vi "PlainTextToVariant (Standard).vi"(11 "String-formatted Value":string) -> (2 "Value Class":T1, 3 "Variant-formatted Value":variant)   [LabVIEW 2013, in "OpenSerializer.lvlib" / "Serializer.PlainText.lvclass"]
uses:
  Serializer.PlainText.lvclass
  Character Class -- Enum.ctl
  <vilib>/LabVIEW Open Source Project/Data Manipulation/Variant/Variant_EmptyCluster.vi
  <vilib>/Utility/GetType.llb/TD_Create Cluster.vi
  <vilib>/LabVIEW Open Source Project/Data Manipulation/Variant/OpenVariant.lvlib
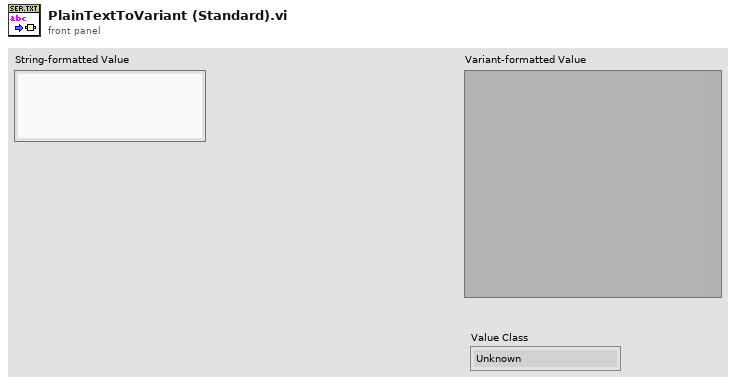
[diagram p1: front panel]
types:
  T1 = typedef "OpenSerializer.lvlib/Serializer.PlainText.lvclass/Character Class -- Enum.ctl" = enum16{"Unknown", "Sign", "Zero", "Integer", "Float", "Complex", "Scientific", "Engineering", "Hexadecimal", "Binary", "Decimal", "Octal", "Unit", "Invalid", "Timestamp", "Boolean", "String", "Path", "null", "cluster", "array"}
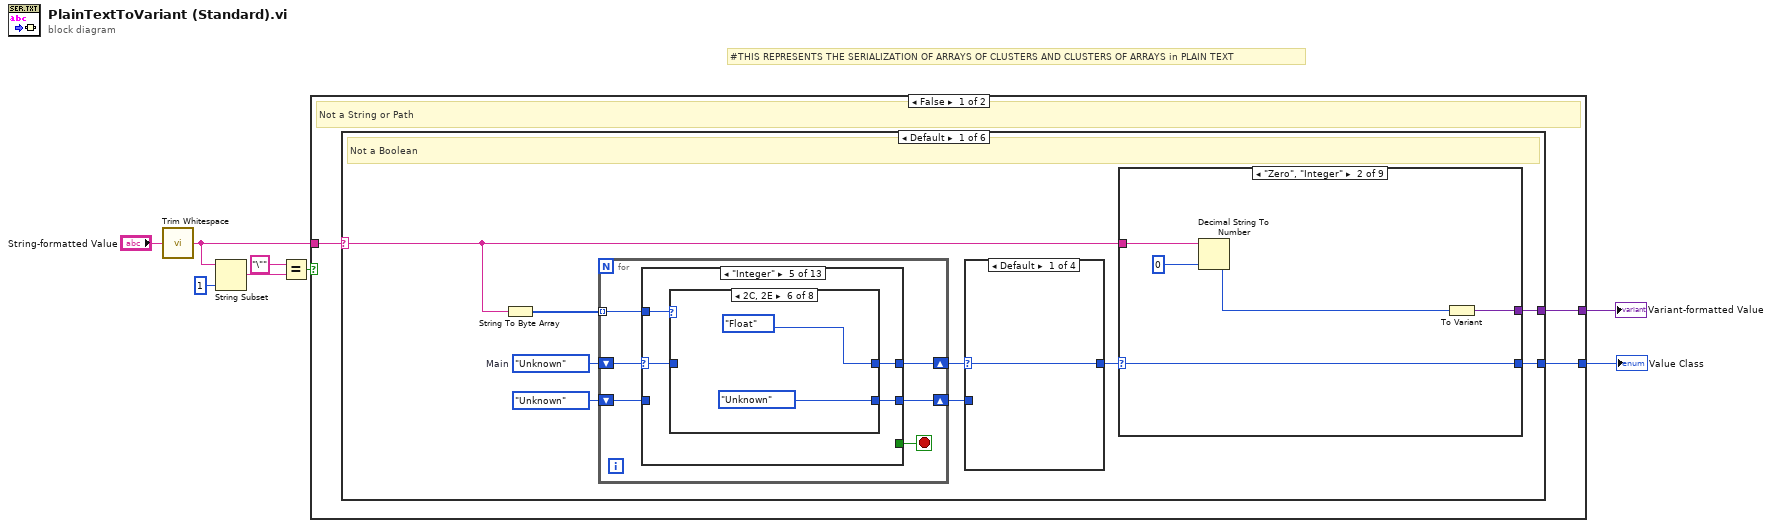
[diagram p0: block diagram]
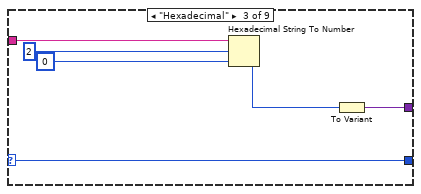
[diagram p3: hidden frame]
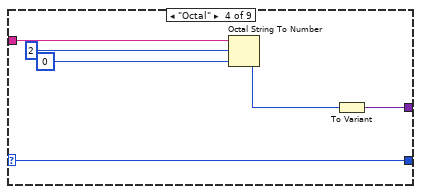
[diagram p4: hidden frame]
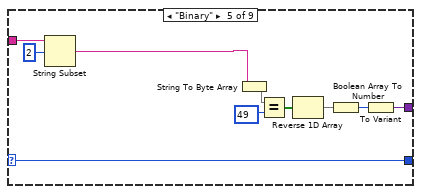
[diagram p5: hidden frame]
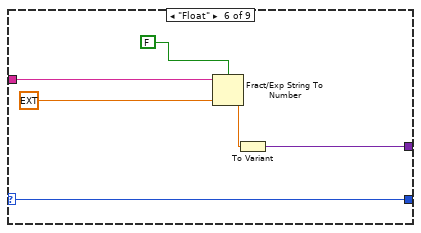
[diagram p6: hidden frame]
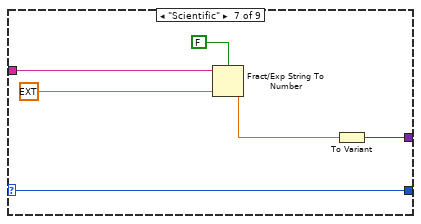
[diagram p7: hidden frame]
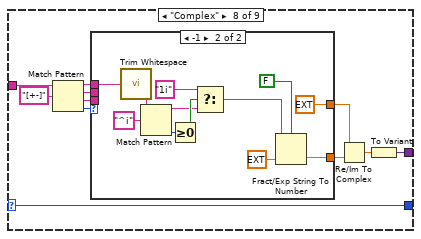
[diagram p8: hidden frame]
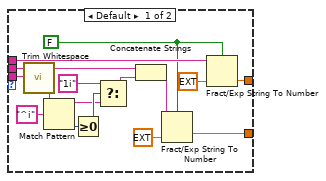
[diagram p9: hidden frame]
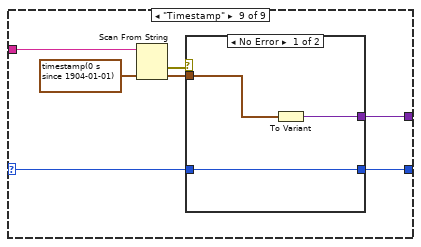
[diagram p10: hidden frame]
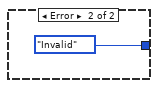
[diagram p11: hidden frame]
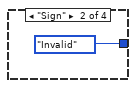
[diagram p12: hidden frame]
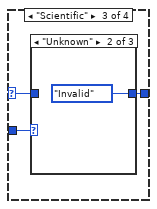
[diagram p13: hidden frame]
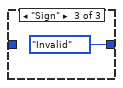
[diagram p15: hidden frame]
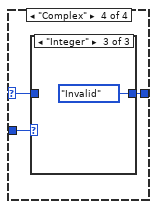
[diagram p16: hidden frame]
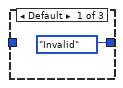
[diagram p17: hidden frame]
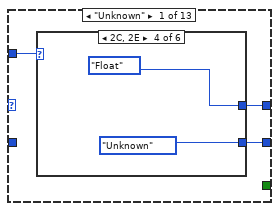
[diagram p19: hidden frame]
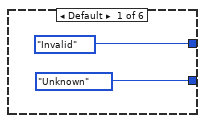
[diagram p20: hidden frame]
diagram:
  # "#THIS REPRESENTS THE SERIALIZATION OF ARRAYS OF CLUSTERS AND CLUSTERS OF ARRAYS in PLAIN TEXT"
  n1 = call <vilib>:"Trim Whitespace.vi"("string"="String-formatted Value") -> ("trimmed string"=w7:string)  [unwired: 1 in]
  n2 = String Subset(string=w7, length (rest)=1 ("length (rest)")) -> (substring=w5:string)  [unwired: 1 in]
  n3 = Equal?(x="\"", y=w5) -> (x = y?=w3:bool)
  n4 = case shown="False" w3 {
    tunnel: w7 -> [w11 w568]
    tunnel: [w10 w576] -> w8
    tunnel: [w9 w569] -> w2
    frame False {
      # "Not a String or Path"
      n5 = case shown="Default" w11 {
        selector: w11 -> [w15 _ _ _ w340 w457]
        tunnel: [w14 w328 w331 w335 w344 w461] -> w10
        tunnel: [w13 Character_Class_--_Enum."Boolean" Character_Class_--_Enum."Boolean" Character_Class_--_Enum."null" w343 w460] -> w9
        frame Default {
          w19 = Character_Class_--_Enum."Unknown"  # Main
          # "Not a Boolean"
          n6 = String To Byte Array(string=w15) -> (unsigned byte array=w20:u8[])
          n7 = for {
            tunnel: w20 -> [w129] mode=indexing
            shift-right: [w128] -> w18
            shift-left: w19 -> [w130]
            shift-right: [w126] -> w17
            shift-left: Character_Class_--_Enum."Unknown" -> [w127]
            stop <- w125 stop-if-true
            n8 = case shown="\"Integer\"" w130 {
              selector: w130 -> [_ w147 w150 w163 w188 w206 w212 w218 w224 w230 w233 w249 w289]
              tunnel: w129 -> [w133 _ w152 w165 w190 w208 w214 w220 w226 _ w235 w251 w291]
              tunnel: [w132 w147 w151 w164 w189 w207 w213 w219 w225 w230 w234 w250 w290] -> w128
              tunnel: w127 -> [_ w146 w148 _ _ _ _ _ _ _ _ w248 w288]
              tunnel: [w131 w146 w149 w162 w187 Character_Class_--_Enum."Unknown" Character_Class_--_Enum."Unknown" Character_Class_--_Enum."Unknown" Character_Class_--_Enum."Unknown" Character_Class_--_Enum."Unknown" w232 w247 w287] -> w126
              tunnel: [_ TRUE _ _ _ _ _ _ _ TRUE _ _ _] -> w125
              frame "Unknown" {
                n9 = case shown="2C, 2E" w133 {
                  tunnel: [Character_Class_--_Enum."Invalid" Character_Class_--_Enum."Sign" Character_Class_--_Enum."Integer" Character_Class_--_Enum."Float" Character_Class_--_Enum."Zero" w144] -> w132
                  tunnel: [Character_Class_--_Enum."Unknown" Character_Class_--_Enum."Unknown" Character_Class_--_Enum."Unknown" Character_Class_--_Enum."Unknown" Character_Class_--_Enum."Unknown" w144] -> w131
                  frame Default {
                  }
                  frame 43, 45 {
                  }
                  frame 49..57 {
                  }
                  frame 44, 46 {
                  }
                  frame 48 {
                  }
                  frame 105 {
                    w144 = Character_Class_--_Enum."Complex"
                  }
                }
              }
              frame "Invalid", Default {
              }
              frame "Sign" {
                n10 = case shown="2C, 2E" w152 {
                  tunnel: [Character_Class_--_Enum."Invalid" w156 Character_Class_--_Enum."Integer" w159 Character_Class_--_Enum."Float"] -> w151
                  tunnel: w150 -> [_ w156 _ _ _]
                  tunnel: [Character_Class_--_Enum."Unknown" w155 Character_Class_--_Enum."Unknown" w159 Character_Class_--_Enum."Unknown"] -> w149
                  tunnel: w148 -> [_ w155 _ _ _]
                  frame Default {
                  }
                  frame 32 {
                    # "space (ignore)"
                  }
                  frame 48..57 {
                  }
                  frame 105 {
                    w159 = Character_Class_--_Enum."Complex"
                  }
                  frame 44, 46 {
                  }
                }
              }
              frame "Zero" {
                n11 = case shown="Default" w165 {
                  tunnel: [Character_Class_--_Enum."Invalid" Character_Class_--_Enum."Integer" w171 Character_Class_--_Enum."Float" Character_Class_--_Enum."Hexadecimal" Character_Class_--_Enum."Binary" Character_Class_--_Enum."Octal" Character_Class_--_Enum."Decimal" w183 w184 Character_Class_--_Enum."Complex"] -> w164
                  tunnel: w163 -> [_ _ w171 _ _ _ _ _ w183 _ _]
                  tunnel: [Character_Class_--_Enum."Unknown" Character_Class_--_Enum."Unknown" Character_Class_--_Enum."Unknown" Character_Class_--_Enum."Unknown" Character_Class_--_Enum."Unknown" Character_Class_--_Enum."Unknown" Character_Class_--_Enum."Unknown" Character_Class_--_Enum."Unknown" Character_Class_--_Enum."Unknown" w184 Character_Class_--_Enum."Unknown"] -> w162
                  frame Default {
                  }
                  frame 49..57 {
                  }
                  frame 48 {
                  }
                  frame 44, 46 {
                  }
                  frame 120 {
                  }
                  frame 98 {
                  }
                  frame 111 {
                  }
                  frame 100 {
                  }
                  frame 32 {
                  }
                  frame 105 {
                    w184 = Character_Class_--_Enum."Complex"
                  }
                  frame 43, 45 {
                  }
                }
              }
              frame "Integer" {
                n12 = case shown="2C, 2E" w190 {
                  tunnel: [Character_Class_--_Enum."Invalid" w193 w194 w196 w198 Character_Class_--_Enum."Float" Character_Class_--_Enum."Complex" Character_Class_--_Enum."Scientific"] -> w189
                  tunnel: w188 -> [_ _ _ w196 w198 _ _ _]
                  tunnel: [Character_Class_--_Enum."Unknown" w193 w194 Character_Class_--_Enum."Unknown" Character_Class_--_Enum."Unknown" Character_Class_--_Enum."Unknown" Character_Class_--_Enum."Unknown" Character_Class_--_Enum."Unknown"] -> w187
                  frame Default {
                  }
                  frame 105 {
                    w193 = Character_Class_--_Enum."Complex"
                  }
                  frame 58 {
                    w194 = Character_Class_--_Enum."Timestamp"
                  }
                  frame 32 {
                  }
                  frame 48..57 {
                  }
                  frame 44, 46 {
                  }
                  frame 43, 45 {
                  }
                  frame 69, 101 {
                  }
                }
              }
              frame "Hexadecimal" {
                n13 = case shown="30..39, 41..46" w208 {
                  tunnel: [Character_Class_--_Enum."Invalid" w210] -> w207
                  tunnel: w206 -> [_ w210]
                  frame Default {
                  }
                  frame 48..57, 65..70 {
                  }
                }
              }
              frame "Decimal" {
                n14 = case shown="30..39" w214 {
                  tunnel: [Character_Class_--_Enum."Invalid" w216] -> w213
                  tunnel: w212 -> [_ w216]
                  frame Default {
                  }
                  frame 48..57 {
                  }
                }
              }
              frame "Octal" {
                n15 = case shown="30..37" w220 {
                  tunnel: [Character_Class_--_Enum."Invalid" w222] -> w219
                  tunnel: w218 -> [_ w222]
                  frame Default {
                  }
                  frame 48..55 {
                  }
                }
              }
              frame "Binary" {
                n16 = case shown="30, 31" w226 {
                  tunnel: [Character_Class_--_Enum."Invalid" w228] -> w225
                  tunnel: w224 -> [_ w228]
                  frame Default {
                  }
                  frame 48, 49 {
                  }
                }
              }
              frame "Timestamp" {
              }
              frame "Float" {
                n17 = case shown="2B, 2D" w235 {
                  tunnel: [Character_Class_--_Enum."Invalid" w239 Character_Class_--_Enum."Scientific" w243 Character_Class_--_Enum."Complex" w246] -> w234
                  tunnel: w233 -> [_ w239 _ w243 _ _]
                  tunnel: [Character_Class_--_Enum."Unknown" Character_Class_--_Enum."Unknown" Character_Class_--_Enum."Unknown" Character_Class_--_Enum."Unknown" Character_Class_--_Enum."Unknown" w246] -> w232
                  frame Default {
                  }
                  frame 48..57 {
                  }
                  frame 69, 101 {
                  }
                  frame 32 {
                  }
                  frame 43, 45 {
                  }
                  frame 105 {
                    w246 = Character_Class_--_Enum."Complex"
                  }
                }
              }
              frame "Scientific" {
                n18 = case shown="2B, 2D" w251 {
                  tunnel: [Character_Class_--_Enum."Invalid" w255 w267 w280] -> w250
                  tunnel: w249 -> [_ w254 w269 w282]
                  tunnel: w248 -> [w252 w256 w268 w281]
                  tunnel: [w252 w257 w270 w283] -> w247
                  frame Default {
                  }
                  frame 49..57 {
                    n19 = case shown="\"Unknown\"" w256 {
                      selector: w256 -> [_ _ _ w263 _]
                      tunnel: [w258 Character_Class_--_Enum."Integer" Character_Class_--_Enum."Integer" w263 Character_Class_--_Enum."Integer"] -> w257
                      tunnel: [w258 w259 w262 w264 w266] -> w255
                      tunnel: w254 -> [_ w259 w262 w264 w266]
                      frame Default {
                        w258 = Character_Class_--_Enum."Invalid"
                      }
                      frame "Sign" {
                      }
                      frame "Zero" {
                      }
                      frame "Integer" {
                      }
                      frame "Unknown" {
                      }
                    }
                  }
                  frame 48 {
                    n20 = case shown="\"Sign\"" w268 {
                      tunnel: [w271 Character_Class_--_Enum."Zero" Character_Class_--_Enum."Zero" Character_Class_--_Enum."Zero" Character_Class_--_Enum."Integer"] -> w270
                      tunnel: w269 -> [_ w272 w274 w276 w278]
                      tunnel: [w271 w272 w274 w276 w278] -> w267
                      frame Default {
                        w271 = Character_Class_--_Enum."Invalid"
                      }
                      frame "Unknown" {
                      }
                      frame "Sign" {
                      }
                      frame "Zero" {
                      }
                      frame "Integer" {
                      }
                    }
                  }
                  frame 43, 45 {
                    n21 = case shown="\"Unknown\"" w281 {
                      tunnel: [w284 Character_Class_--_Enum."Sign"] -> w283
                      tunnel: w282 -> [_ w285]
                      tunnel: [w284 w285] -> w280
                      frame Default {
                        w284 = Character_Class_--_Enum."Invalid"
                      }
                      frame "Unknown" {
                      }
                    }
                  }
                }
              }
              frame "Complex" {
                n22 = case shown="2C, 2E" w291 {
                  selector: w291 -> [_ _ _ w306 _]
                  tunnel: [w292 w294 w297 w309 w318] -> w290
                  tunnel: w289 -> [_ w294 w295 w307 w316]
                  tunnel: w288 -> [_ w293 w298 w310 w319]
                  tunnel: [w292 w293 w296 w308 w317] -> w287
                  frame Default {
                    w292 = Character_Class_--_Enum."Invalid"
                  }
                  frame 32 {
                  }
                  frame 48..57 {
                    n23 = case shown="Default" w298 {
                      selector: w298 -> [_ _ w302 w304]
                      tunnel: [w299 w301 w303 w305] -> w297
                      tunnel: [w299 Character_Class_--_Enum."Integer" w302 w304] -> w296
                      tunnel: w295 -> [_ w301 w303 w305]
                      frame Default {
                        w299 = Character_Class_--_Enum."Invalid"
                      }
                      frame "Unknown" {
                      }
                      frame "Integer" {
                      }
                      frame "Float" {
                      }
                    }
                  }
                  frame 44, 46 {
                    n24 = case shown="\"Unknown\"" w310 {
                      tunnel: [w311 w313 w315] -> w309
                      tunnel: [w311 Character_Class_--_Enum."Float" Character_Class_--_Enum."Float"] -> w308
                      tunnel: w307 -> [_ w313 w315]
                      tunnel: w306 -> [_ _ _]
                      frame Default {
                        w311 = Character_Class_--_Enum."Invalid"
                      }
                      frame "Unknown" {
                      }
                      frame "Integer" {
                      }
                    }
                  }
                  frame 105 {
                    n25 = case shown="\"Float\"" w319 {
                      tunnel: [w320 w322 w324 w326] -> w318
                      tunnel: [w320 Character_Class_--_Enum."Complex" Character_Class_--_Enum."Complex" Character_Class_--_Enum."Complex"] -> w317
                      tunnel: w316 -> [_ w322 w324 w326]
                      frame Default {
                        w320 = Character_Class_--_Enum."Invalid"
                      }
                      frame "Unknown" {
                      }
                      frame "Integer" {
                      }
                      frame "Float" {
                      }
                    }
                  }
                }
              }
            }
          }
          n26 = case shown="Default" w18 {
            selector: w18 -> [w111 _ w113 w119]
            tunnel: w17 -> [_ _ w115 w121]
            tunnel: [w111 Character_Class_--_Enum."Invalid" w114 w120] -> w16
            frame Default {
            }
            frame "Sign" {
            }
            frame "Scientific" {
              n27 = case shown="\"Unknown\"" w115 {
                tunnel: [w116 Character_Class_--_Enum."Invalid" Character_Class_--_Enum."Invalid"] -> w114
                tunnel: w113 -> [w116 _ _]
                frame Default {
                }
                frame "Unknown" {
                }
                frame "Sign" {
                }
              }
            }
            frame "Complex" {
              n28 = case shown="\"Integer\"" w121 {
                tunnel: [Character_Class_--_Enum."Invalid" w123 Character_Class_--_Enum."Invalid" ("Main")] -> w120
                tunnel: w119 -> [_ w123 _]
                frame Default {
                }
                frame "Complex" {
                }
                frame "Integer" {
                }
              }
            }
          }
          n29 = case shown="\"Zero\", \"Integer\"" w16 {
            selector: w16 -> [w21 w22 w27 w33 w39 w50 w56 w70 w100]
            tunnel: w15 -> [_ w26 w32 w38 w47 w54 w60 w66 w106]
            tunnel: [_ w23 w29 w35 w48 w51 w57 w71 w103] -> w14
            tunnel: [w21 w22 w27 w33 w39 w50 w56 w70 w101] -> w13
            frame Default {
            }
            frame "Zero", "Integer" {
              n30 = Decimal String To Number(string=w26, default (0L)=i64 0 ("default (0 I32)")) -> (number=w24:i64)  [unwired: 1 in, 1 out]
              n31 = To Variant(anything=w24) -> (Variant=w23:variant)
            }
            frame "Hexadecimal" {
              n32 = Hexadecimal String To Number(string=w32, offset=2, default (0uL)=i64 0 ("default (0 I32)")) -> (number=w30:i64)  [unwired: 1 out]
              n33 = To Variant(anything=w30) -> (Variant=w29:variant)
            }
            frame "Octal" {
              n34 = Octal String To Number(2:i64 0 ("default (0 I32)"), 3:2 ("offset"), 4:w38) -> (0:w36:i64)  [unwired: 1 out]
              n35 = To Variant(anything=w36) -> (Variant=w35:variant)
            }
            frame "Binary" {
              n36 = String Subset(string=w47, offset (0)=2) -> (substring=w45:string)  [unwired: 1 in]
              n37 = String To Byte Array(string=w45) -> (unsigned byte array=w43:u8[])
              n38 = Equal?(x=w43, y=u8 49 ("offset (0)")) -> (x = y?=w42:bool[])
              n39 = Reverse 1D Array(array=w42) -> (reversed array=w40:bool[])
              n40 = Boolean Array To Number(Boolean array=w40) -> (number=w44:u32)
              n41 = To Variant(anything=w44) -> (Variant=w48:variant)
            }
            frame "Float" {
              n42 = Fract/Exp String To Number(use system decimal point (T)=FALSE, string=w54, default (0 dbl)=ext 0.0 ("default (0 I32)")) -> (number=w52:ext)  [unwired: 1 in, 1 out]
              n43 = To Variant(anything=w52) -> (Variant=w51:variant)
            }
            frame "Scientific" {
              n44 = Fract/Exp String To Number(use system decimal point (T)=FALSE, string=w60, default (0 dbl)=ext 0.0 ("default (0 I32)")) -> (number=w58:ext)  [unwired: 1 in, 1 out]
              n45 = To Variant(anything=w58) -> (Variant=w57:variant)
            }
            frame "Complex" {
              n46 = Match Pattern(string=w66, regular expression="[+-]") -> (before substring=w63:string, match substring=w61:string, after substring=w62:string, offset past match=w67:i32)  [unwired: 1 in]
              n47 = case shown="-1" w67 {
                tunnel: [w84 ext 0.0 ("default (0 DBL)")] -> w64
                tunnel: [w86 w97] -> w65
                tunnel: w63 -> [w83 w90]
                tunnel: w62 -> [w74 _]
                tunnel: w61 -> [w77 _]
                frame Default {
                  w72 = FALSE ("use system decimal point (T)")
                  n48 = call <vilib>:"Trim Whitespace.vi"("string"=w74) -> ("trimmed string"=w75:string)  [unwired: 1 in]
                  n49 = Match Pattern(string=w75, regular expression="^i") -> (before substring=w80:string, offset past match=w82:i32)  [unwired: 1 in, 2 out]
                  n50 = Greater Or Equal To 0?(x=w82) -> (x >= 0?=w81:bool)
                  n51 = Select(t="1i", s=w81, f=w80) -> (s? t:f=w78:string)
                  n52 = Concatenate Strings(w77, w78) -> (w76:string)
                  n53 = Fract/Exp String To Number(use system decimal point (T)=w72, string=w76, default (0 dbl)=ext 0.0 ("default (0 DBL)")) -> (number=w86:ext)  [unwired: 1 in, 1 out]
                  n54 = Fract/Exp String To Number(use system decimal point (T)=w72, string=w83, default (0 dbl)=ext 0.0 ("default (0 DBL)")) -> (number=w84:ext)  [unwired: 1 in, 1 out]
                }
                frame -1 {
                  n55 = call <vilib>:"Trim Whitespace.vi"("string"=w90) -> ("trimmed string"=w92:string)  [unwired: 1 in]
                  n56 = Match Pattern(string=w92, regular expression="^i") -> (before substring=w94:string, offset past match=w96:i32)  [unwired: 1 in, 2 out]
                  n57 = Greater Or Equal To 0?(x=w96) -> (x >= 0?=w95:bool)
                  n58 = Select(t="1i", s=w95, f=w94) -> (s? t:f=w89:string)
                  n59 = Fract/Exp String To Number(use system decimal point (T)=FALSE, string=w89, default (0 dbl)=ext 0.0 ("default (0 DBL)")) -> (number=w97:ext)  [unwired: 1 in, 1 out]
                }
              }
              n60 = Re/Im To Complex(1:w65, 2:w64) -> (0:w69:cxt)
              n61 = To Variant(anything=w69) -> (Variant=w71:variant)
            }
            frame "Timestamp" {
              n62 = Scan From String(input string=w106, default 1=timestamp(0 s since 1904-01-01)) -> (error out=w102:errorcluster, output 1=w104:timestamp)  [unwired: 3 in, 2 out]
              n63 = case shown="No Error" w102 {
                tunnel: w104 -> [w109 _]
                tunnel: [w108 _] -> w103
                tunnel: [w107 Character_Class_--_Enum."Invalid"] -> w101
                tunnel: w100 -> [w107 _]
                frame No Error {
                  n64 = To Variant(anything=w109) -> (Variant=w108:variant)
                }
                frame Error {
                }
              }
            }
          }
        }
        frame "true" {
          # "BOOLEAN (TRUE)"
          n65 = To Variant(anything=TRUE) -> (Variant=w328:variant)
        }
        frame "false" {
          # "BOOLEAN (FALSE)"
          n66 = To Variant(anything=FALSE) -> (Variant=w331:variant)
        }
        frame "null" {
          # "null"
          n67 = To Variant(anything=variant ("variant")) -> (Variant=w335:variant)
        }
        frame "{".."{~" {
          # "cluster"
          n68 = String Length(string=w340) -> (length=w342:i32)
          n69 = Subtract(x=w342, y=1) -> (x-y=w336:i32)
          n70 = String Subset(string=w340, offset (0)=w336) -> (substring=w338:string)  [unwired: 1 in]
          n71 = Equal?(x="}", y=w338) -> (x = y?=w337:bool)
          n72 = case shown="True" w337 {
            tunnel: [w353 w452] -> w344
            tunnel: [Character_Class_--_Enum."cluster" Character_Class_--_Enum."Invalid"] -> w343
            tunnel: w340 -> [w359 _]
            tunnel: w336 -> [w357 _]
            frame True {
              n73 = Decrement(x=w357) -> (x-1=w356:i32)
              n74 = String Subset(string=w359, offset (0)=1, length (rest)=w356) -> (substring=w355:string)
              n75 = call <vilib>:"Trim Whitespace.vi"("string"=w355) -> ("trimmed string"=w350:string)  [unwired: 1 in]
              n76 = String Length(string=w350) -> (length=w351:i32)
              n77 = for {
                N: w351 -> [_]
                shift-right: [w364] -> w347
                shift-left: string[] [] -> [w365]
                tunnel: w350 -> [w370]
                shift-right: [w363] -> w348
                shift-left: "" -> [w366]
                shift-right: [w361] -> _
                shift-left: Character_Class_--_Enum."Unknown" -> [w362]
                i -> [w369]
                n78 = String Subset(string=w370, offset (0)=w369, length (rest)=1 ("offset (0)")) -> (substring=w367:string)
                n79 = case shown="Default" w367 {
                  selector: w367 -> [w374 w377 w395 w407 w421 w435]
                  tunnel: w366 -> [w373 w382 w396 w408 w422 w436]
                  tunnel: w365 -> [w375 w381 w398 w410 w424 w438]
                  tunnel: [w375 w380 w398 w410 w424 w438] -> w364
                  tunnel: [w372 w379 w394 w406 w420 w434] -> w363
                  tunnel: w362 -> [w371 w378 w397 w409 w423 w437]
                  tunnel: [w371 w376 w393 w405 w419 w433] -> w361
                  frame Default {
                    n80 = Concatenate Strings(w373, w374) -> (w372:string)
                  }
                  frame "," {
                    n81 = case shown="\"Unknown\", Default" w378 {
                      selector: w378 -> [w383 w388]
                      tunnel: w382 -> [w387 w391]
                      tunnel: w381 -> [w386 w392]
                      tunnel: [w385 w392] -> w380
                      tunnel: ["" w389] -> w379
                      tunnel: w377 -> [_ w390]
                      tunnel: [w383 w388] -> w376
                      frame "Unknown", Default {
                        n82 = Build Array (concatenate)(w386, w387) -> (w385:string[])
                      }
                      frame "cluster", "array" {
                        n83 = Concatenate Strings(w391, w390) -> (w389:string)
                      }
                    }
                  }
                  frame "{" {
                    n84 = case shown="Default" w397 {
                      selector: w397 -> [_ w401]
                      tunnel: w396 -> [_ w404]
                      tunnel: w395 -> [w399 w403]
                      tunnel: [w399 w402] -> w394
                      tunnel: [Character_Class_--_Enum."cluster" w401] -> w393
                      frame Default {
                      }
                      frame "cluster" {
                        n85 = Concatenate Strings(w404, w403) -> (w402:string)
                      }
                    }
                  }
                  frame "}" {
                    n86 = case shown="\"cluster\"" w409 {
                      selector: w409 -> [w411 _]
                      tunnel: w408 -> [w414 w416]
                      tunnel: w407 -> [w413 w417]
                      tunnel: [w412 w415] -> w406
                      tunnel: [w411 Character_Class_--_Enum."Unknown"] -> w405
                      frame Default {
                        n87 = Concatenate Strings(w414, w413) -> (w412:string)
                      }
                      frame "cluster" {
                        n88 = Concatenate Strings(w416, w417) -> (w415:string)
                      }
                    }
                  }
                  frame "[" {
                    n89 = case shown="Default" w423 {
                      tunnel: w422 -> [w428 w430]
                      tunnel: w421 -> [w427 w431]
                      tunnel: [w426 w429] -> w420
                      tunnel: [Character_Class_--_Enum."array" Character_Class_--_Enum."array"] -> w419
                      frame Default {
                        n90 = Concatenate Strings(w428, w427) -> (w426:string)
                      }
                      frame "cluster" {
                        n91 = Concatenate Strings(w430, w431) -> (w429:string)
                      }
                    }
                  }
                  frame "]" {
                    n92 = case shown="\"array\"" w437 {
                      selector: w437 -> [w439 _]
                      tunnel: w436 -> [w442 w444]
                      tunnel: w435 -> [w441 w445]
                      tunnel: [w440 w443] -> w434
                      tunnel: [w439 Character_Class_--_Enum."Unknown"] -> w433
                      frame Default {
                        n93 = Concatenate Strings(w442, w441) -> (w440:string)
                      }
                      frame "array" {
                        n94 = Concatenate Strings(w444, w445) -> (w443:string)
                      }
                    }
                  }
                }
              }
              n95 = Build Array (concatenate)(w347, w348) -> (w346:string[])
              n96 = for {
                tunnel: w346 -> [w449] mode=indexing
                tunnel: [w447] -> w354 mode=indexing
                n97 = call <vilib>:"Trim Whitespace.vi"("string"=w449) -> ("trimmed string"=w448:string)  [unwired: 1 in]
                n98 = call "PlainTextToVariant (Standard).vi"("String-formatted Value"=w448) -> ("Variant-formatted Value"=w447:variant)  [unwired: 9 in, 1 out]
              }
              n99 = call <vilib>:"Variant_BuildClusterFromElementArray.vi"("Elements"=w354) -> ("Cluster"=w353:variant)  [unwired: 10 in]
            }
            frame False {
              n100 = To Variant(anything=variant ("variant")) -> (Variant=w452:variant)
            }
          }
        }
        frame "[".."[~" {
          # "array"
          n101 = String Length(string=w457) -> (length=w459:i32)
          n102 = Subtract(x=w459, y=1) -> (x-y=w453:i32)
          n103 = String Subset(string=w457, offset (0)=w453) -> (substring=w455:string)  [unwired: 1 in]
          n104 = Equal?(x="]", y=w455) -> (x = y?=w454:bool)
          n105 = case shown="True" w454 {
            tunnel: [w465 w567] -> w461
            tunnel: [Character_Class_--_Enum."array" Character_Class_--_Enum."Invalid"] -> w460
            tunnel: w457 -> [w463 _]
            tunnel: w453 -> [w475 _]
            frame True {
              # "#THIS IS UPDATED AS WELL\nto support undefined array input"
              n106 = Decrement(x=w475) -> (x-1=w474:i32)
              n107 = String Subset(string=w463, offset (0)=1, length (rest)=w474) -> (substring=w462:string)
              n108 = call <vilib>:"Trim Whitespace.vi"("string"=w462) -> ("trimmed string"=w471:string)  [unwired: 1 in]
              n109 = String Length(string=w471) -> (length=w472:i32)
              n110 = for {
                N: w472 -> [_]
                shift-right: [w481] -> w468
                shift-left: string[] [] -> [w482]
                tunnel: w471 -> [w487]
                shift-right: [w480] -> w469
                shift-left: "" -> [w483]
                shift-right: [w478] -> _
                shift-left: Character_Class_--_Enum."Unknown" -> [w479]
                i -> [w486]
                n111 = String Subset(string=w487, offset (0)=w486, length (rest)=1 ("offset (0)")) -> (substring=w484:string)
                n112 = case shown="\"]\"" w484 {
                  selector: w484 -> [w491 w494 w512 w524 w536 w550]
                  tunnel: w483 -> [w490 w499 w513 w525 w537 w551]
                  tunnel: w482 -> [w492 w498 w515 w527 w539 w553]
                  tunnel: [w492 w497 w515 w527 w539 w553] -> w481
                  tunnel: [w489 w496 w511 w523 w535 w549] -> w480
                  tunnel: w479 -> [w488 w495 w514 w526 w538 w552]
                  tunnel: [w488 w493 w510 w522 w534 w548] -> w478
                  frame Default {
                    n113 = Concatenate Strings(w490, w491) -> (w489:string)
                  }
                  frame "," {
                    n114 = case shown="\"cluster\"" w495 {
                      selector: w495 -> [w500 w505]
                      tunnel: w499 -> [w504 w508]
                      tunnel: w498 -> [w503 w509]
                      tunnel: [w502 w509] -> w497
                      tunnel: ["" w506] -> w496
                      tunnel: w494 -> [_ w507]
                      tunnel: [w500 w505] -> w493
                      frame "Unknown", Default {
                        n115 = Build Array (concatenate)(w503, w504) -> (w502:string[])
                      }
                      frame "cluster" {
                        n116 = Concatenate Strings(w508, w507) -> (w506:string)
                      }
                    }
                  }
                  frame "[" {
                    n117 = case shown="\"array\"" w514 {
                      selector: w514 -> [_ w518]
                      tunnel: w513 -> [_ w521]
                      tunnel: w512 -> [w516 w520]
                      tunnel: [w516 w519] -> w511
                      tunnel: [Character_Class_--_Enum."array" w518] -> w510
                      frame Default {
                      }
                      frame "array" {
                        n118 = Concatenate Strings(w521, w520) -> (w519:string)
                      }
                    }
                  }
                  frame "{" {
                    n119 = case shown="Default" w526 {
                      selector: w526 -> [_ w530]
                      tunnel: w525 -> [_ w533]
                      tunnel: w524 -> [w528 w532]
                      tunnel: [w528 w531] -> w523
                      tunnel: [Character_Class_--_Enum."cluster" w530] -> w522
                      frame Default {
                      }
                      frame "cluster" {
                        n120 = Concatenate Strings(w533, w532) -> (w531:string)
                      }
                    }
                  }
                  frame "]" {
                    n121 = case shown="\"array\"" w538 {
                      selector: w538 -> [w540 _]
                      tunnel: w537 -> [w543 w545]
                      tunnel: w536 -> [w542 w546]
                      tunnel: [w541 w544] -> w535
                      tunnel: [w540 Character_Class_--_Enum."Unknown"] -> w534
                      frame Default {
                        n122 = Concatenate Strings(w543, w542) -> (w541:string)
                      }
                      frame "array" {
                        n123 = Concatenate Strings(w545, w546) -> (w544:string)
                      }
                    }
                  }
                  frame "}" {
                    n124 = case shown="\"cluster\"" w552 {
                      selector: w552 -> [w554 _]
                      tunnel: w551 -> [w557 w559]
                      tunnel: w550 -> [w556 w560]
                      tunnel: [w555 w558] -> w549
                      tunnel: [w554 Character_Class_--_Enum."Unknown"] -> w548
                      frame Default {
                        n125 = Concatenate Strings(w557, w556) -> (w555:string)
                      }
                      frame "cluster" {
                        n126 = Concatenate Strings(w559, w560) -> (w558:string)
                      }
                    }
                  }
                }
              }
              n127 = Build Array (concatenate)(w468, w469) -> (w467:string[])
              n128 = for {
                tunnel: w467 -> [w564] mode=indexing
                tunnel: [w562] -> w464 mode=indexing
                n129 = call <vilib>:"Trim Whitespace.vi"("string"=w564) -> ("trimmed string"=w563:string)  [unwired: 1 in]
                n130 = call "PlainTextToVariant (Standard).vi"("String-formatted Value"=w563) -> ("Variant-formatted Value"=w562:variant)  [unwired: 9 in, 1 out]
              }
              n131 = call <vilib>:"Variant_BuildArrayFromElementArray.vi"("Elements"=w464) -> ("Output Array"=w465:variant)  [unwired: 9 in, 1 out]
            }
            frame False {
              n132 = To Variant(anything=variant ("variant")) -> (Variant=w567:variant)
            }
          }
        }
      }
    }
    frame True {
      # "String or Path"
      n133 = String Length(string=w568) -> (length=w575:i32)
      n134 = Decrement(x=w575) -> (x-1=w571:i32)
      n135 = String Subset(string=w568, offset (0)=w571, length (rest)=1 ("length (rest)")) -> (substring=w572:string)
      n136 = Equal?(x=w572, y="\"" ("x")) -> (x = y?=w570:bool)
      n137 = case shown="True" w570 {
        tunnel: [_ w579] -> w576
        tunnel: w568 -> [_ w590]
        tunnel: w571 -> [_ w589]
        tunnel: [Character_Class_--_Enum."Invalid" w578] -> w569
        frame False {
        }
        frame True {
          n138 = Decrement(x=w589) -> (x-1=w588:i32)
          n139 = String Subset(string=w590, offset (0)=1, length (rest)=w588) -> (substring=w580:string)
          n140 = String Subset(string=w580, length (rest)=1 ("length (rest)")) -> (substring=w586:string)  [unwired: 1 in]
          n141 = Equal?(x="/", y=w586) -> (x = y?=w584:bool)
          n142 = Select(t=u8 50 ("Type"), s=w584, f=u8 48 ("Type")) -> (s? t:f=w581:u8)
          n143 = case shown="32" w581 {
            tunnel: [w595 w598] -> w579
            tunnel: w580 -> [w594 w596]
            tunnel: [Character_Class_--_Enum."Path" Character_Class_--_Enum."String"] -> w578
            frame 50 {
              # "PATH (0x32)"
              n144 = call "Common Path to Specific Path.vi"("common path"=w594) -> ("specific path"=w593:path)  [unwired: 10 in]
              n145 = To Variant(anything=w593) -> (Variant=w595:variant)
            }
            frame 48, Default {
              # "STRING (0x30)"
              n146 = To Variant(anything=w596) -> (Variant=w598:variant)
            }
          }
        }
      }
    }
  }
  "Variant-formatted Value" <- w8
  "Value Class" <- w2
